vi "Dialog abilita potenza.vi"() -> (2 "Abilita?":bool caption="Time has Elapsed")   [LabVIEW 2019]
panel:
  out "Boolean":bool
  out "concatenated string":string
  in  "Annulla":bool
  in  "ABILITA POTENZA":bool
  out "Boolean 2":bool
  # "CHIUDERE IL TELERUTTORE DI POTENZA?"
  # "1- ASSICURARSI CHE I CAVI DI POTENZA \n    SIANO IN SICUREZZA\n\n2- ASSICURARSI CHE IL CARTER DI PROTEZIONE\n    SIA CHIUSO\n\n3- VERIFICARE DI AVER CONNESSO LA PRESA ILME CORRETTA PER LE MISURE ELETTRICHE"
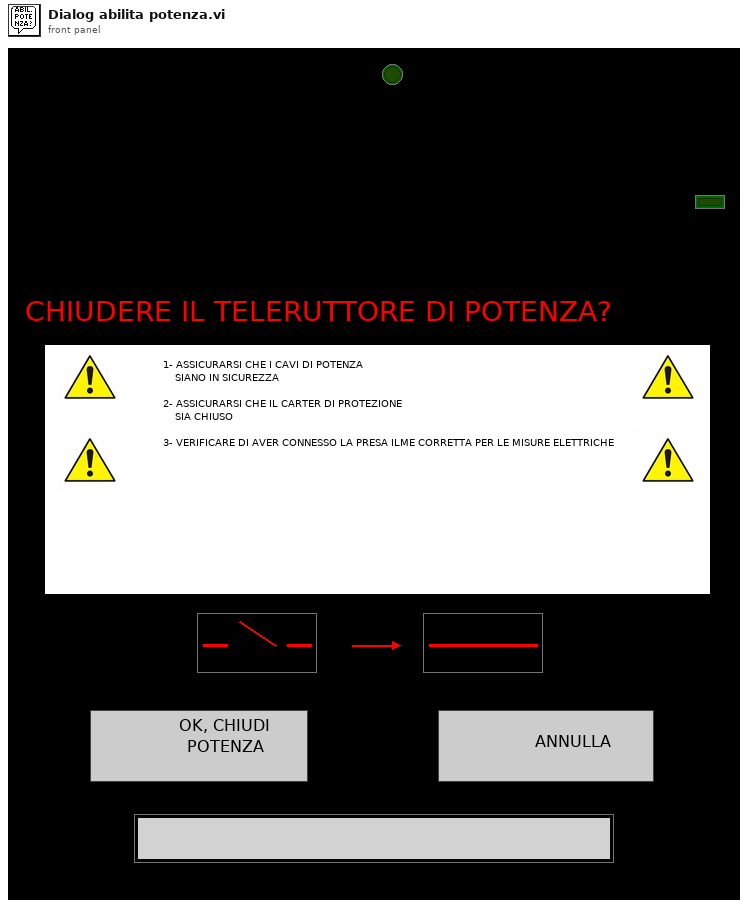
[diagram p1: front panel]
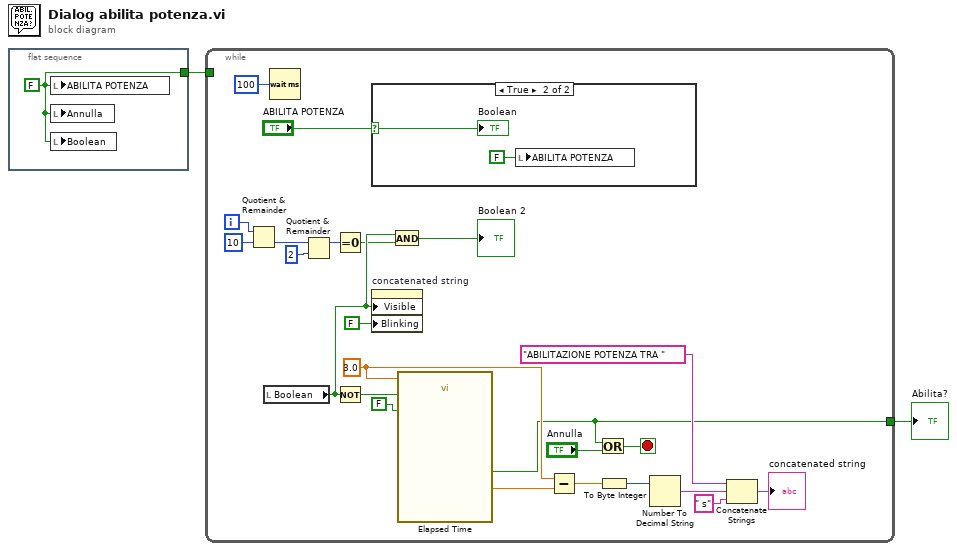
[diagram p0: block diagram]
diagram:
  n1 = flat-sequence {
    tunnel: [w3] -> w2
    frame #0 {
      w3 = FALSE ("ABILITA POTENZA")
      n2 = local write "ABILITA POTENZA"(w3) -> ()
      n3 = local write "Annulla"(w3) -> ()
      n4 = local write "Boolean"(w3) -> ()
    }
  }
  n5 = while {
    tunnel: w2 -> [_]
    tunnel: [w4] -> w1
    i -> [w10]
    stop <- w24 stop-if-true
    w22 = 3.0 ("Time Target (s)")
    n6 = Quotient & Remainder(x=w10, y=10) -> (floor(x/y)=w6:i32)  [unwired: 1 out]
    n7 = local read "Boolean"() -> (w12:bool)
    n8 = Wait (ms)(milliseconds to wait=u32 100) -> ()  [unwired: 1 out]
    n9 = Quotient & Remainder(x=w6, y=2) -> (x-y*floor(x/y)=w5:i32)  [unwired: 1 out]
    n10 = Equal To 0?(x=w5) -> (x = 0?=w7:bool)
    n11 = Not(x=w12) -> (.not. x?=w26:bool)
    n12 = case shown="True" "ABILITA POTENZA" {
      selector: "ABILITA POTENZA" -> [_ w29]
      frame False {
      }
      frame True {
        n13 = local write "ABILITA POTENZA"(FALSE ("ABILITA POTENZA")) -> ()
        "Boolean" <- w29
      }
    }
    n14 = property on="concatenated string" class="Str"("Visible"=w12, "Blinking"=FALSE) -> ()  [unwired: 2 in, 2 out]
    n15 = And(x=w12, y=w7) -> (x .and. y?=→"Boolean 2":bool)
    n16 = call "Elapsed Time"("Time Target (s)"=w22, "Reset"=w26, "Auto Reset"=FALSE) -> ("Elapsed Time (s)"=w21:dbl, "Time has Elapsed"=w4:bool)  [unwired: 9 in, 6 out]
    n17 = Subtract(x=w22, y=w21) -> (x-y=w18:dbl)
    n18 = Or(x=w4, y="Annulla") -> (x .or. y?=w24:bool)
    n19 = To Byte Integer(number=w18) -> (8bit integer=w15:i8)
    n20 = Number To Decimal String(number=w15) -> (decimal integer string=w17:string)  [unwired: 1 in]
    n21 = Concatenate Strings("ABILITAZIONE POTENZA TRA ", w17, " s" ("string")) -> (→"concatenated string":string)
  }
  "Abilita?" <- w1
